vi "Read Sample offset DVR.vi"(11 "Waveform Session in":refnum<class "Waveform Session.lvclass">) -> (2 "Sample offset":refnum<data-value>, 3 "Waveform Session out":refnum<class "Waveform Session.lvclass">)   [LabVIEW 2020, in "NI_VS Custom Device Waveform API.lvlib" / "Waveform Session.lvclass"]
uses:
  Waveform Session.lvclass
  Waveform Session.lvclass/Waveform Session.ctl
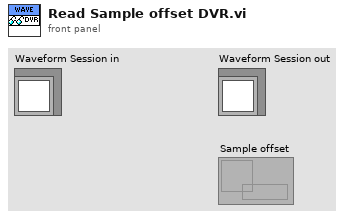
[diagram p1: front panel]
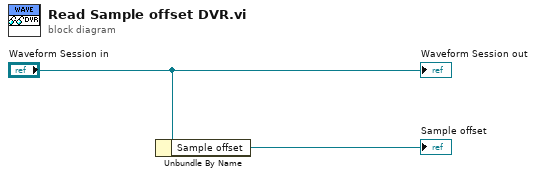
[diagram p0: block diagram]
diagram:
  n1 = Unbundle By Name("Waveform Session in") -> ("Sample offset"=→"Sample offset":refnum<data-value>)
  "Waveform Session out" <- "Waveform Session in"
